vi "test UXX Writes to Source.vi"(8 "error in (no error)":errorcluster, 11 "TestCase in":refnum<class "Parameter Setting.lvclass">) -> (0 "error out":errorcluster, 3 "TestCase out":refnum<class "Parameter Setting.lvclass">)   [LabVIEW 2017, in "Deterministic Error Tests.lvlib" / "Parameter Setting.lvclass"]
uses:
  Parameter Setting.lvclass
  Parameter Setting.lvclass/Parameter Setting.ctl
  Source/VIs/Source.Write.Scalar.Base10 (U64).vi
  Source/VIs/Source.Write.Scalar.Base10 (U32).vi
  Source/VIs/Source.Write.Scalar.Base10 (U16).vi
  Source/VIs/Source.Write.Scalar.Base10 (U8).vi
  <vilib>/addons/_JKI Toolkits/VI Tester/TestCase.llb/TestCase.lvclass
  Source/Static Error Handling.lvlib
  C:/Program Files (x86)/National Instruments/LabVIEW 2017/vi.lib/addons/_JKI Toolkits/VI Tester/TestCase.llb/TestCase.lvclass
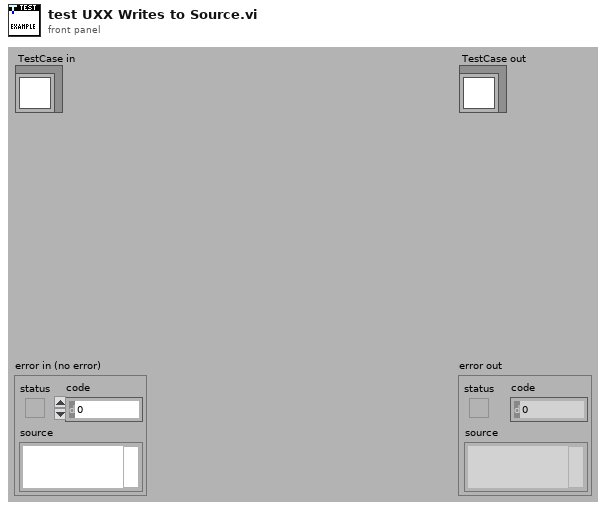
[diagram p1: front panel]
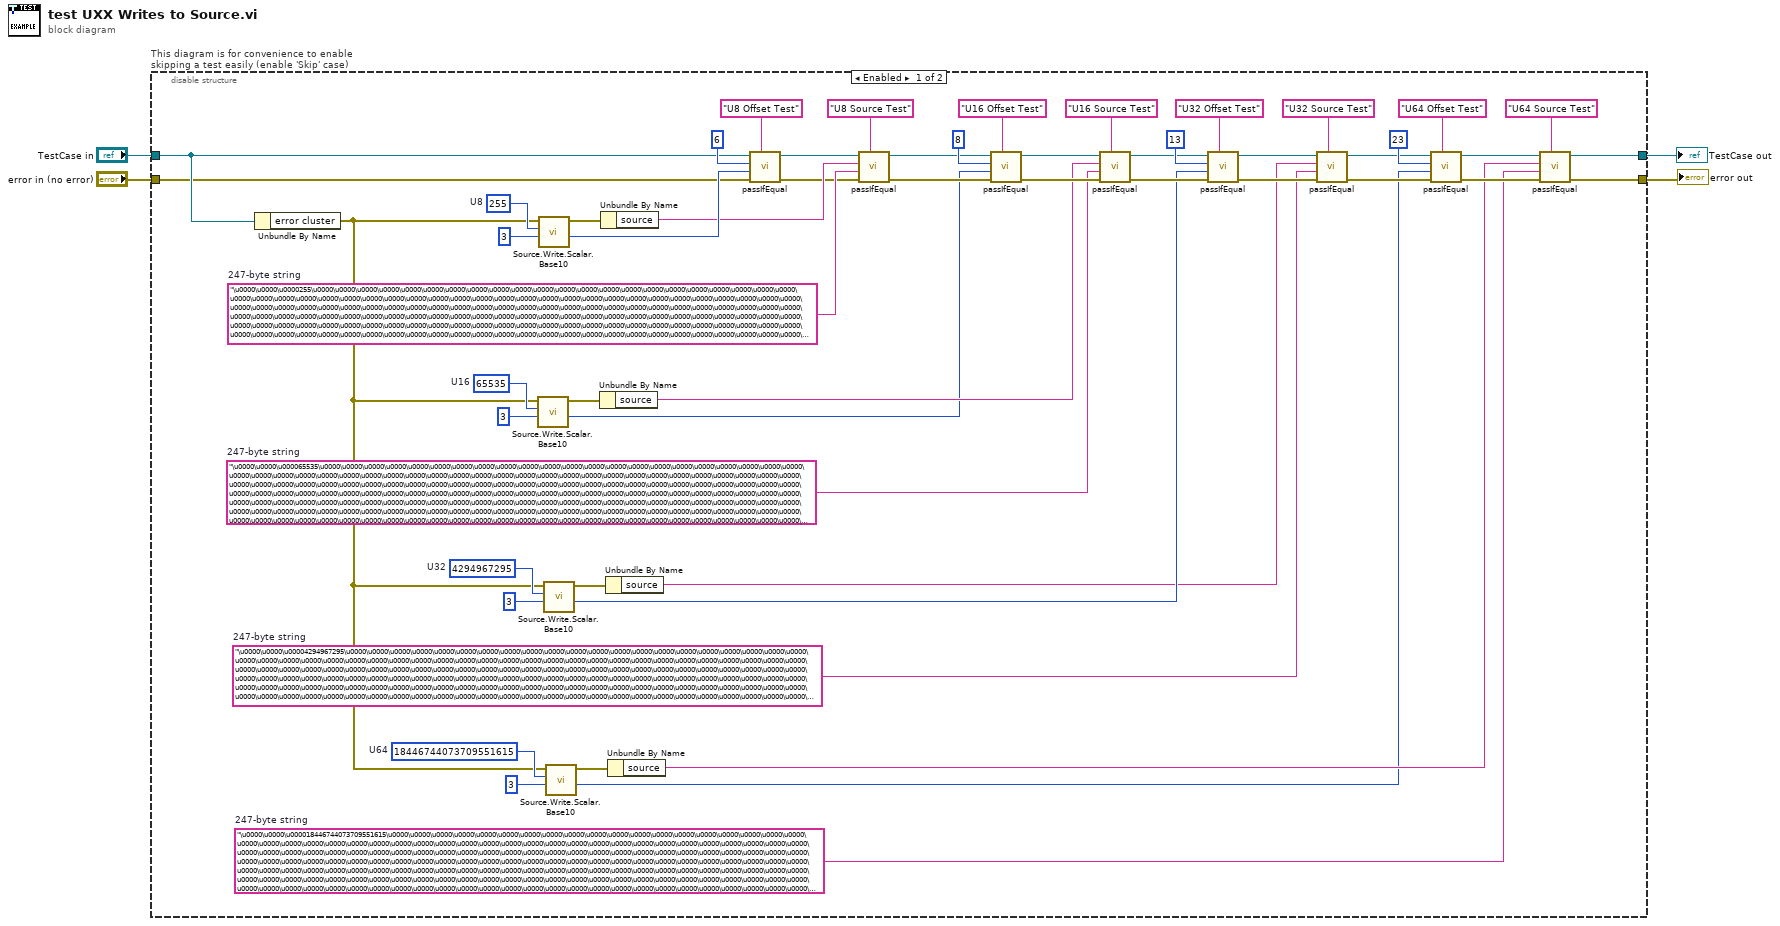
[diagram p0: block diagram]
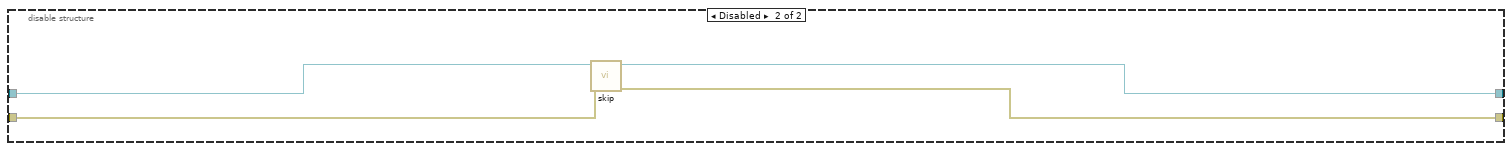
[diagram p2: hidden frame]
diagram:
  n1 = disable-structure "This diagram is for convenience to enable skipping a test easily (enable 'Skip' case)" shown="Enabled" {
    disable-tunnel: "TestCase in" -> [w8 w63]
    disable-tunnel: [w6 w61] -> w1
    disable-tunnel: [w5 w62] -> w3
    disable-tunnel: "error in (no error)" -> [w7 w60]
    frame Enabled {
      w10 = "\u0000\u0000\u000018446744073709551615\u0000\u0000\u0000\u0000\u0000\u0000\u0000\u0000\u0000\u0000\u0000\u0000\u0000\u0000\u0000\u0000\u0000\u0000\u0000\u0000\u0000\u0000\u0000\u0000\u0000\u0000\u0000\u0000\u0000\u0000\u0000\u0000\u0000\u0000\u0000\u0000\u0000\u0000\u0000\u0000\u0000\u0000\u0000\u0000\u0000\u0000\u0000\u0000\u0000\u0000\u0000\u0000\u0000\u0000\u0000\u0000\u0000\u0000\u0000\u0000\u0000\u0000\u0000\u0000\u0000\u0000\u0000\u0000\u0000\u0000\u0000\u0000\u0000\u0000\u0000\u0000\u0000\u0000\u0000\u0000\u0000\u0000\u0000\u0000\u0000\u0000\u0000\u0000\u0000\u0000\u0000\u0000\u0000\u0000\u0000\u0000\u0000\u0000\u0000\u0000\u0000\u0000\u0000\u0000\u0000\u0000\u0000\u0000\u0000\u0000\u0000\u0000\u0000\u0000\u0000\u0000\u0000\u0000\u0000\u0000\u0000\u0000\u0000\u0000\u0000\u0000\u0000\u0000\u0000\u0000\u0000\u0000\u0000\u0000\u0000\u0000\u0000\u0000\u0000\u0000\u0000\u0000\u0000\u0000\u0000\u0000\u0000\u0000\u0000\u0000\u0000\u0000\u0000\u0000\u0000\u0000\u0000\u0000\u0000\u0000\u0000\u0000\u0000\u0000\u0000\u0000\u0000\u0000\u0000\u0000\u0000\u0000\u0000\u0000\u0000\u0000\u0000\u0000\u0000\u0000\u0000\u0000\u0000\u0000\u0000\u0000\u0000\u0000\u0000\u0000\u0000\u0000\u0000\u0000\u0000\u0000\u0000\u0000\u0000\u0000\u0000\u0000\u0000\u0000\u0000\u0000\u0000\u0000\u0000\u0000\u0000\u0000\u0000\u0000\u0000\u0000\u0000\u0000\u0000\u0000\u0000\u0000\u0000\u0000"  # 247-byte string
      w15 = u64 18446744073709551615  # U64
      w23 = "\u0000\u0000\u00004294967295\u0000\u0000\u0000\u0000\u0000\u0000\u0000\u0000\u0000\u0000\u0000\u0000\u0000\u0000\u0000\u0000\u0000\u0000\u0000\u0000\u0000\u0000\u0000\u0000\u0000\u0000\u0000\u0000\u0000\u0000\u0000\u0000\u0000\u0000\u0000\u0000\u0000\u0000\u0000\u0000\u0000\u0000\u0000\u0000\u0000\u0000\u0000\u0000\u0000\u0000\u0000\u0000\u0000\u0000\u0000\u0000\u0000\u0000\u0000\u0000\u0000\u0000\u0000\u0000\u0000\u0000\u0000\u0000\u0000\u0000\u0000\u0000\u0000\u0000\u0000\u0000\u0000\u0000\u0000\u0000\u0000\u0000\u0000\u0000\u0000\u0000\u0000\u0000\u0000\u0000\u0000\u0000\u0000\u0000\u0000\u0000\u0000\u0000\u0000\u0000\u0000\u0000\u0000\u0000\u0000\u0000\u0000\u0000\u0000\u0000\u0000\u0000\u0000\u0000\u0000\u0000\u0000\u0000\u0000\u0000\u0000\u0000\u0000\u0000\u0000\u0000\u0000\u0000\u0000\u0000\u0000\u0000\u0000\u0000\u0000\u0000\u0000\u0000\u0000\u0000\u0000\u0000\u0000\u0000\u0000\u0000\u0000\u0000\u0000\u0000\u0000\u0000\u0000\u0000\u0000\u0000\u0000\u0000\u0000\u0000\u0000\u0000\u0000\u0000\u0000\u0000\u0000\u0000\u0000\u0000\u0000\u0000\u0000\u0000\u0000\u0000\u0000\u0000\u0000\u0000\u0000\u0000\u0000\u0000\u0000\u0000\u0000\u0000\u0000\u0000\u0000\u0000\u0000\u0000\u0000\u0000\u0000\u0000\u0000\u0000\u0000\u0000\u0000\u0000\u0000\u0000\u0000\u0000\u0000\u0000\u0000\u0000\u0000\u0000\u0000\u0000\u0000\u0000\u0000\u0000\u0000\u0000\u0000\u0000\u0000\u0000\u0000\u0000\u0000\u0000\u0000\u0000\u0000\u0000"  # 247-byte string
      w26 = u32 4294967295  # U32
      w36 = "\u0000\u0000\u000065535\u0000\u0000\u0000\u0000\u0000\u0000\u0000\u0000\u0000\u0000\u0000\u0000\u0000\u0000\u0000\u0000\u0000\u0000\u0000\u0000\u0000\u0000\u0000\u0000\u0000\u0000\u0000\u0000\u0000\u0000\u0000\u0000\u0000\u0000\u0000\u0000\u0000\u0000\u0000\u0000\u0000\u0000\u0000\u0000\u0000\u0000\u0000\u0000\u0000\u0000\u0000\u0000\u0000\u0000\u0000\u0000\u0000\u0000\u0000\u0000\u0000\u0000\u0000\u0000\u0000\u0000\u0000\u0000\u0000\u0000\u0000\u0000\u0000\u0000\u0000\u0000\u0000\u0000\u0000\u0000\u0000\u0000\u0000\u0000\u0000\u0000\u0000\u0000\u0000\u0000\u0000\u0000\u0000\u0000\u0000\u0000\u0000\u0000\u0000\u0000\u0000\u0000\u0000\u0000\u0000\u0000\u0000\u0000\u0000\u0000\u0000\u0000\u0000\u0000\u0000\u0000\u0000\u0000\u0000\u0000\u0000\u0000\u0000\u0000\u0000\u0000\u0000\u0000\u0000\u0000\u0000\u0000\u0000\u0000\u0000\u0000\u0000\u0000\u0000\u0000\u0000\u0000\u0000\u0000\u0000\u0000\u0000\u0000\u0000\u0000\u0000\u0000\u0000\u0000\u0000\u0000\u0000\u0000\u0000\u0000\u0000\u0000\u0000\u0000\u0000\u0000\u0000\u0000\u0000\u0000\u0000\u0000\u0000\u0000\u0000\u0000\u0000\u0000\u0000\u0000\u0000\u0000\u0000\u0000\u0000\u0000\u0000\u0000\u0000\u0000\u0000\u0000\u0000\u0000\u0000\u0000\u0000\u0000\u0000\u0000\u0000\u0000\u0000\u0000\u0000\u0000\u0000\u0000\u0000\u0000\u0000\u0000\u0000\u0000\u0000\u0000\u0000\u0000\u0000\u0000\u0000\u0000\u0000\u0000\u0000\u0000\u0000\u0000\u0000\u0000\u0000\u0000\u0000\u0000\u0000\u0000\u0000\u0000\u0000"  # 247-byte string
      w48 = u16 65535  # U16
      w50 = "\u0000\u0000\u0000255\u0000\u0000\u0000\u0000\u0000\u0000\u0000\u0000\u0000\u0000\u0000\u0000\u0000\u0000\u0000\u0000\u0000\u0000\u0000\u0000\u0000\u0000\u0000\u0000\u0000\u0000\u0000\u0000\u0000\u0000\u0000\u0000\u0000\u0000\u0000\u0000\u0000\u0000\u0000\u0000\u0000\u0000\u0000\u0000\u0000\u0000\u0000\u0000\u0000\u0000\u0000\u0000\u0000\u0000\u0000\u0000\u0000\u0000\u0000\u0000\u0000\u0000\u0000\u0000\u0000\u0000\u0000\u0000\u0000\u0000\u0000\u0000\u0000\u0000\u0000\u0000\u0000\u0000\u0000\u0000\u0000\u0000\u0000\u0000\u0000\u0000\u0000\u0000\u0000\u0000\u0000\u0000\u0000\u0000\u0000\u0000\u0000\u0000\u0000\u0000\u0000\u0000\u0000\u0000\u0000\u0000\u0000\u0000\u0000\u0000\u0000\u0000\u0000\u0000\u0000\u0000\u0000\u0000\u0000\u0000\u0000\u0000\u0000\u0000\u0000\u0000\u0000\u0000\u0000\u0000\u0000\u0000\u0000\u0000\u0000\u0000\u0000\u0000\u0000\u0000\u0000\u0000\u0000\u0000\u0000\u0000\u0000\u0000\u0000\u0000\u0000\u0000\u0000\u0000\u0000\u0000\u0000\u0000\u0000\u0000\u0000\u0000\u0000\u0000\u0000\u0000\u0000\u0000\u0000\u0000\u0000\u0000\u0000\u0000\u0000\u0000\u0000\u0000\u0000\u0000\u0000\u0000\u0000\u0000\u0000\u0000\u0000\u0000\u0000\u0000\u0000\u0000\u0000\u0000\u0000\u0000\u0000\u0000\u0000\u0000\u0000\u0000\u0000\u0000\u0000\u0000\u0000\u0000\u0000\u0000\u0000\u0000\u0000\u0000\u0000\u0000\u0000\u0000\u0000\u0000\u0000\u0000\u0000\u0000\u0000\u0000\u0000\u0000\u0000\u0000\u0000\u0000\u0000\u0000\u0000\u0000\u0000\u0000\u0000\u0000\u0000"  # 247-byte string
      w53 = u8 255  # U8
      n2 = Unbundle By Name(w8) -> ("error cluster"=w12:errorcluster)
      n3 = call-poly "Source.Write.Scalar.Base10.vi"("offset"=3, "value"=w48, "error in"=w12) -> ("new offset"=w37:i32, "error out"=w46:errorcluster)  [unwired: 7 in]
      n4 = call-poly "Source.Write.Scalar.Base10.vi"("offset"=3, "value"=w53, "error in"=w12) -> ("new offset"=w52:i32, "error out"=w55:errorcluster)  [unwired: 7 in]
      n5 = call-poly "Source.Write.Scalar.Base10.vi"("offset"=3, "value"=w26, "error in"=w12) -> ("new offset"=w25:i32, "error out"=w28:errorcluster)  [unwired: 7 in]
      n6 = call-poly "Source.Write.Scalar.Base10.vi"("offset"=3, "value"=w15, "error in"=w12) -> ("new offset"=w9:i32, "error out"=w13:errorcluster)  [unwired: 7 in]
      n7 = Unbundle By Name(w46) -> ("source"=w38:string)
      n8 = Unbundle By Name(w55) -> ("source"=w51:string)
      n9 = Unbundle By Name(w28) -> ("source"=w24:string)
      n10 = Unbundle By Name(w13) -> ("source"=w11:string)
      n11 = call-dynamic "passIfEqual.vi"("custom report message (\"\")"="U8 Offset Test" ("custom report message (\"\")"), "error in (no error)"=w7, "y"=w52, "x"=6 ("offset"), "TestCase in"=w8) -> ("error out"=w49:errorcluster, "TestCase out"=w56:refnum<class "Parameter Setting.lvclass">)  [unwired: 5 in]
      n12 = call-dynamic "passIfEqual.vi"("custom report message (\"\")"="U8 Source Test" ("custom report message (\"\")"), "error in (no error)"=w49, "y"=w50, "x"=w51, "TestCase in"=w56) -> ("error out"=w39:errorcluster, "TestCase out"=w40:refnum<class "Parameter Setting.lvclass">)  [unwired: 5 in]
      n13 = call-dynamic "passIfEqual.vi"("custom report message (\"\")"="U16 Offset Test" ("custom report message (\"\")"), "error in (no error)"=w39, "y"=w37, "x"=8 ("offset"), "TestCase in"=w40) -> ("error out"=w45:errorcluster, "TestCase out"=w44:refnum<class "Parameter Setting.lvclass">)  [unwired: 5 in]
      n14 = call-dynamic "passIfEqual.vi"("custom report message (\"\")"="U16 Source Test" ("custom report message (\"\")"), "error in (no error)"=w45, "y"=w36, "x"=w38, "TestCase in"=w44) -> ("error out"=w29:errorcluster, "TestCase out"=w30:refnum<class "Parameter Setting.lvclass">)  [unwired: 5 in]
      n15 = call-dynamic "passIfEqual.vi"("custom report message (\"\")"="U32 Offset Test" ("custom report message (\"\")"), "error in (no error)"=w29, "y"=w25, "x"=13 ("offset"), "TestCase in"=w30) -> ("error out"=w31:errorcluster, "TestCase out"=w32:refnum<class "Parameter Setting.lvclass">)  [unwired: 5 in]
      n16 = call-dynamic "passIfEqual.vi"("custom report message (\"\")"="U32 Source Test" ("custom report message (\"\")"), "error in (no error)"=w31, "y"=w23, "x"=w24, "TestCase in"=w32) -> ("error out"=w16:errorcluster, "TestCase out"=w17:refnum<class "Parameter Setting.lvclass">)  [unwired: 5 in]
      n17 = call-dynamic "passIfEqual.vi"("custom report message (\"\")"="U64 Offset Test" ("custom report message (\"\")"), "error in (no error)"=w16, "y"=w9, "x"=23 ("offset"), "TestCase in"=w17) -> ("error out"=w22:errorcluster, "TestCase out"=w21:refnum<class "Parameter Setting.lvclass">)  [unwired: 5 in]
      n18 = call-dynamic "passIfEqual.vi"("custom report message (\"\")"="U64 Source Test" ("custom report message (\"\")"), "error in (no error)"=w22, "y"=w10, "x"=w11, "TestCase in"=w21) -> ("error out"=w5:errorcluster, "TestCase out"=w6:refnum<class "Parameter Setting.lvclass">)  [unwired: 5 in]
    }
    frame Disabled {
      # "skip test result while test is under development"
      n19 = call <vilib>:"skip.vi"("error in (no error)"=w60, "TestCase in"=w63) -> ("error out"=w62:errorcluster, "TestCase out"=w61:refnum<class "Parameter Setting.lvclass">)  [unwired: 8 in]
    }
  }
  "error out" <- w3
  "TestCase out" <- w1
